vi "Show_raw.00.vi"(3 "t":i32(slide) scale=0.0..1.0, 4 "z":i32(slide) scale=0.0..60.0, 5 "file (use dialog)":path) -> (0 "data 4d":dbl[][][][](array[numeric]), 1 "data 3d":dbl[][][](array[numeric]), 2 "data 2d":dbl[][](array[numeric]))   [LabVIEW 2014]
uses:
  <vilib>/picture/picture.llb/Draw True-Color Pixmap.vi
panel:
  in  "color":enum16{"gray", "color"}(ring)
  in  "Bright":dbl(knob)=512.0 scale=-500.0..500.0
  out "pixel size":sgl[](array[numeric])
  in  "Constrast":dbl(knob)=512.0 scale=0.0..2000.0
  in  "State":bool
  out "2D Picture":picture
  in  "Zoom Factor":sgl=5.0
  out "size(s) 3":i32[](array[numeric])
  out "datatype":string
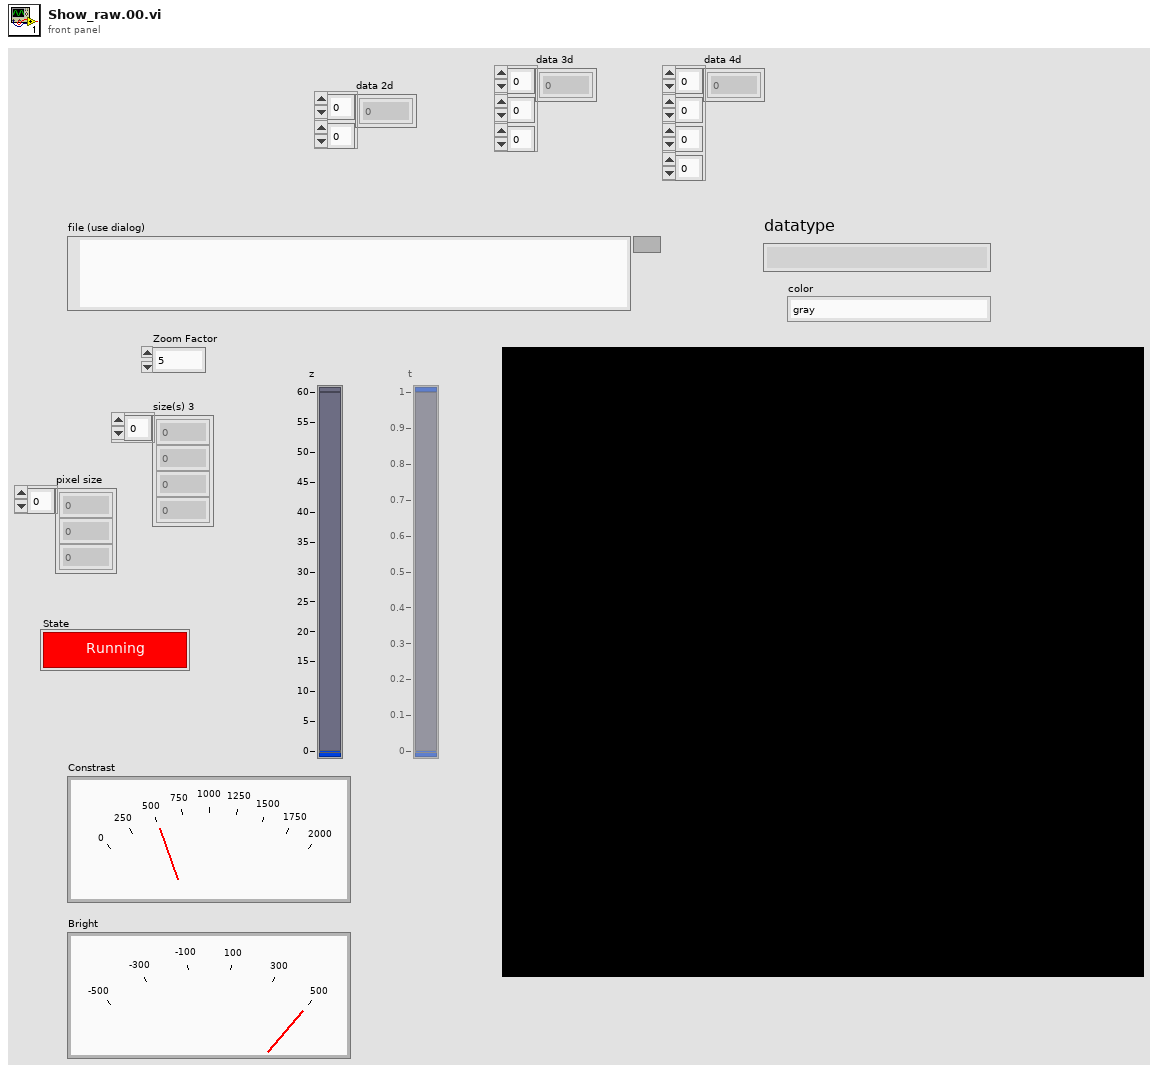
[diagram p1: front panel]
types:
  T1 = enum8{"Enabled", "Disabled", "Disabled and Grayed Out"}
  T2 = typedef "head_data.ctl" = cluster{"hdr size":i32, "dim":i32[], "data bit size":i32, "datatype":string, "pixel size ":sgl[], "voxel offset":sgl, "range of calibration values-max,min":sgl[], " pixel values- max, min":sgl[], "slice orientation":u16}
  T3 = enum32{"Invalid", "Standard", "Closed", "Hidden", "Minimized", "Maximized"}
  T4 = typedef "imagedata.ctl" = cluster{"image type":i32, "image depth":i32, "image":u8[], "mask":u8[], "colors":u32[], "Rectangle":cluster{"left":i16, "top":i16, "right":i16, "bottom":i16}}
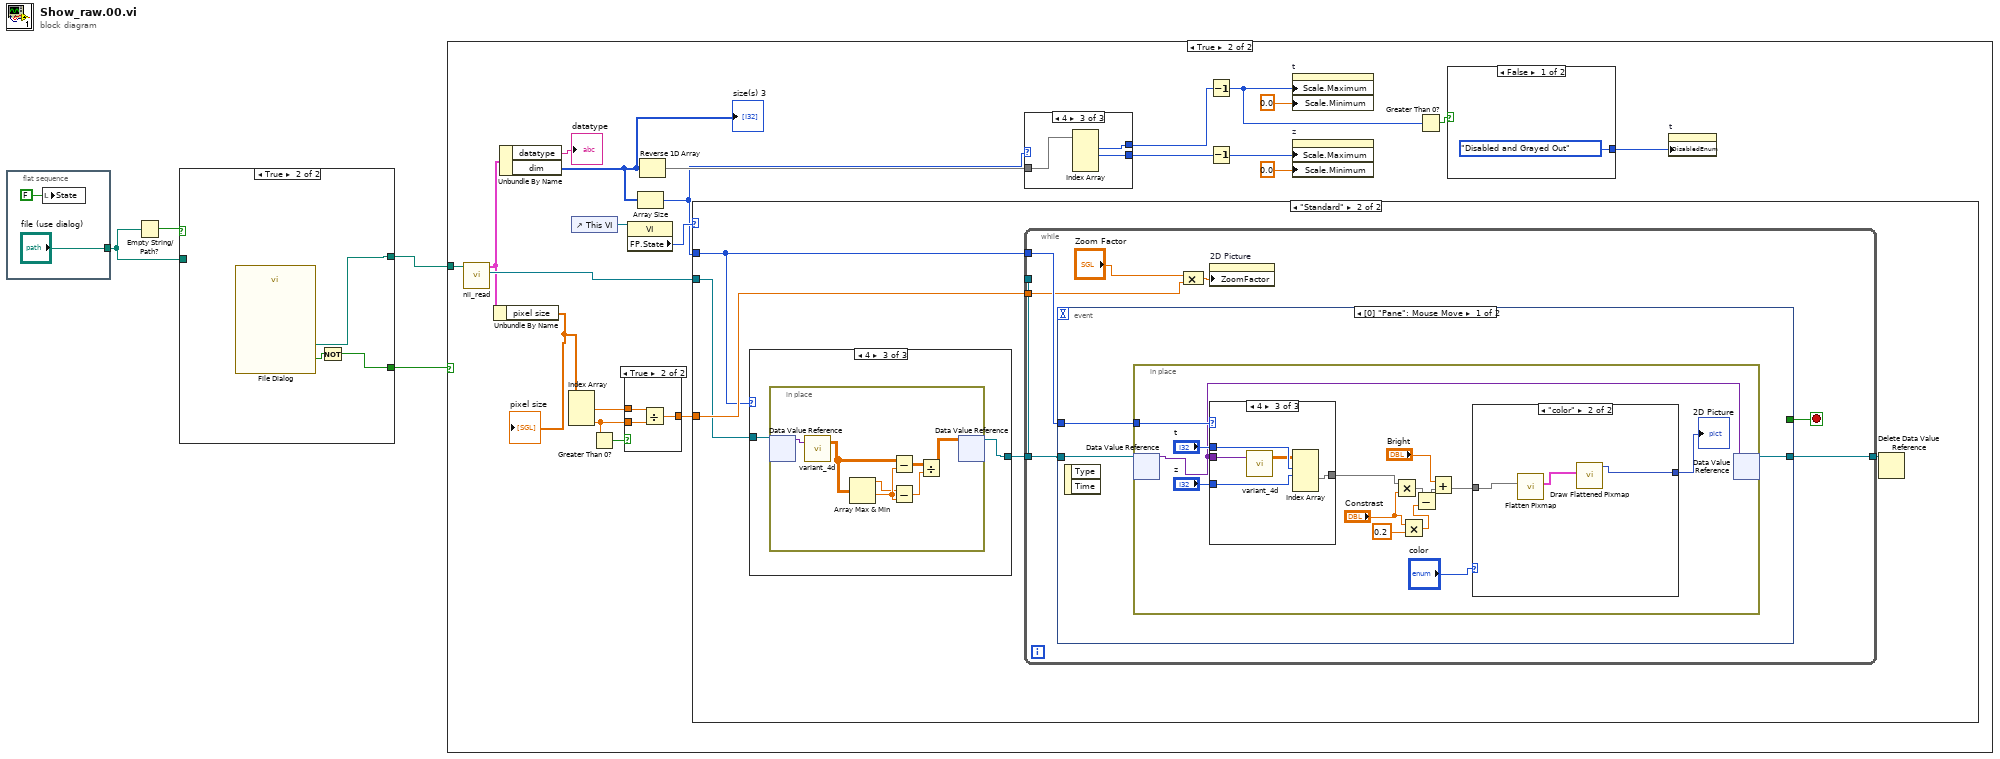
[diagram p0: block diagram]
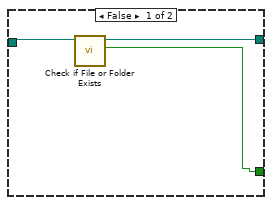
[diagram p2: hidden frame]
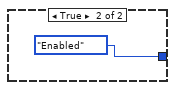
[diagram p4: hidden frame]
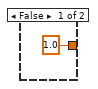
[diagram p5: hidden frame]
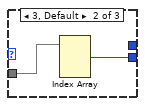
[diagram p7: hidden frame]
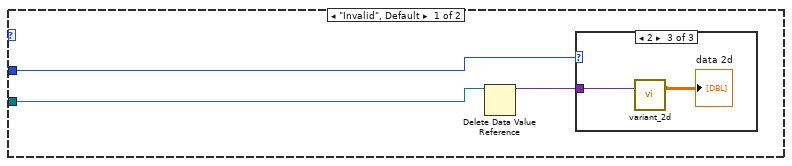
[diagram p8: hidden frame]
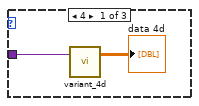
[diagram p9: hidden frame]
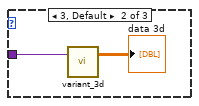
[diagram p10: hidden frame]
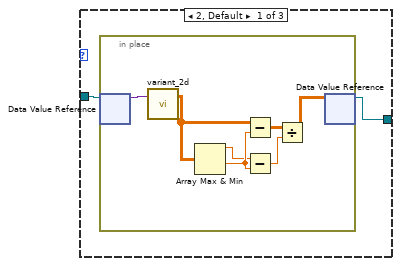
[diagram p11: hidden frame]
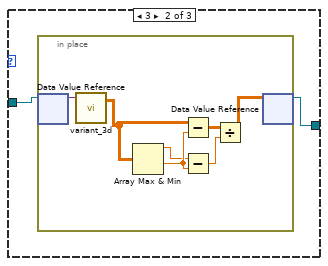
[diagram p12: hidden frame]
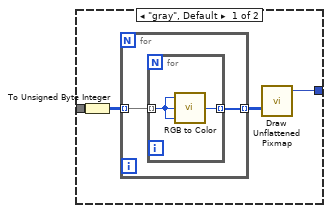
[diagram p13: hidden frame]
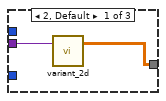
[diagram p14: hidden frame]
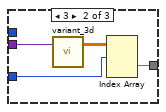
[diagram p15: hidden frame]
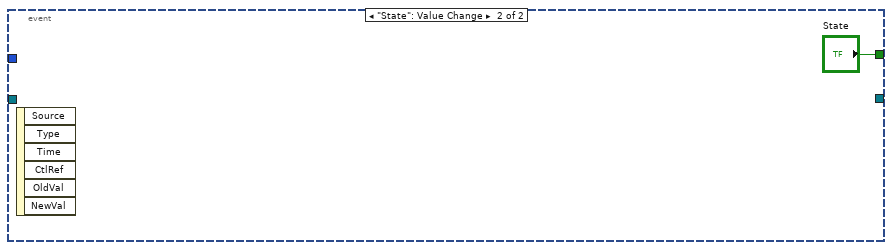
[diagram p16: hidden frame]
diagram:
  n1 = flat-sequence {
    tunnel: ["file (use dialog)"] -> w4
    frame #0 {
      n2 = local write "State"(FALSE ("stop")) -> ()
    }
  }
  n3 = Empty String/Path?(string/path=w4) -> (empty?=w3:bool)
  n4 = case shown="True" w3 {
    tunnel: w4 -> [w9 _]
    tunnel: [w7 w12] -> w1
    tunnel: [w8 w10] -> w2
    frame False {
      n5 = call <vilib>:"Check if File or Folder Exists.vi"("path"=w9) -> ("file or folder exists?"=w7:bool, "dup path"=w8:path)  [unwired: 8 in, 1 out]
    }
    frame True {
      n6 = call "File Dialog"() -> ("selected path"=w10:path, "cancelled"=w11:bool)  [unwired: 12 in, 2 out]
      n7 = Not(x=w11) -> (.not. x?=w12:bool)
    }
  }
  n8 = case shown="True" w1 {
    tunnel: w2 -> [_ w29]
    frame False {
    }
    frame True {
      n9 = call "nii_read.vi"("file (use dialog)"=w29) -> ("data value reference"=w32:refnum<data-value>, "Data"=w22:T2)  [unwired: 6 in, 3 out]
      n10 = Unbundle By Name(w22) -> ("pixel size"=w21:sgl[])
      "pixel size" <- w21
      n11 = Unbundle By Name(w22) -> ("datatype"=→"datatype":string, "dim"=w16:i32[])
      "size(s) 3" <- w16
      n12 = Index Array(array=w21) -> (element #1=w20:sgl, element #3=w19:sgl)  [unwired: 3 in, 1 out]
      n13 = control-ref of="This VI"() -> (w33:refnum<vi>)
      n14 = Greater Than 0?(x=w19) -> (x > 0?=w18:bool)
      n15 = case shown="True" w18 {
        tunnel: w19 -> [_ w38]
        tunnel: w20 -> [_ w40]
        tunnel: [sgl 1.0 w39] -> w17
        frame False {
        }
        frame True {
          n16 = Divide(x=w40, y=w38) -> (x/y=w39:sgl)
        }
      }
      n17 = property class="VI"(reference=w33) -> ("FP.State"=w31:T3)  [unwired: 1 in, 2 out]
      n18 = Array Size(array=w16) -> (size(s)=w26:i32)
      n19 = Reverse 1D Array(array=w16) -> (reversed array=w30:i32[])
      n20 = case shown="\"Standard\"" w31 {
        tunnel: w32 -> [w48 w56]
        tunnel: w26 -> [w47 w57]
        tunnel: w17 -> [_ w59]
        frame "Invalid", Default {
          n21 = Delete Data Value Reference(data value reference=w48) -> (data value=w46:variant)  [unwired: 1 in, 1 out]
          n22 = case shown="2" w47 {
            tunnel: w46 -> [w50 w52 w54]
            frame 4 {
              n23 = call "variant_4d.vi"("variant"=w50) -> ("data"=→"data 4d":dbl[][][][])  [unwired: 2 in]
            }
            frame 3, Default {
              n24 = call "variant_3d.vi"("variant"=w52) -> ("data"=→"data 3d":dbl[][][])  [unwired: 2 in]
            }
            frame 2 {
              n25 = call "variant_2d.vi"("variant"=w54) -> ("data"=→"data 2d":dbl[][])  [unwired: 2 in]
            }
          }
        }
        frame "Standard" {
          n26 = case shown="4" w57 {
            tunnel: w56 -> [w61 w70 w79]
            tunnel: [w60 w69 w78] -> w55
            frame 2, Default {
              n27 = in-place {
                n28 = in-place-dvr #1(w61) -> (w63:variant)  [unwired: 1 out]
                n29 = call "variant_2d.vi"("variant"=w63) -> ("data"=w64:dbl[][])  [unwired: 2 in]
                n30 = Array Max & Min(array=w64) -> (max value=w65:dbl, min value=w66:dbl)  [unwired: 2 out]
                n31 = Subtract(x=w64, y=w66) -> (x-y=w68:dbl[][])
                n32 = Subtract(x=w65, y=w66) -> (x-y=w67:dbl)
                n33 = Divide(x=w68, y=w67) -> (x/y=w62:dbl[][])
                n34 = in-place-dvr #1(w62) -> (w60:refnum<data-value>)  [unwired: 1 out]
              }
            }
            frame 3 {
              n35 = in-place {
                n36 = in-place-dvr #2(w70) -> (w72:variant)  [unwired: 1 out]
                n37 = call "variant_3d.vi"("variant"=w72) -> ("data"=w71:dbl[][][])  [unwired: 2 in]
                n38 = Array Max & Min(array=w71) -> (max value=w74:dbl, min value=w75:dbl)  [unwired: 2 out]
                n39 = Subtract(x=w71, y=w75) -> (x-y=w77:dbl[][][])
                n40 = Subtract(x=w74, y=w75) -> (x-y=w76:dbl)
                n41 = Divide(x=w77, y=w76) -> (x/y=w73:dbl[][][])
                n42 = in-place-dvr #2(w73) -> (w69:refnum<data-value>)  [unwired: 1 out]
              }
            }
            frame 4 {
              n43 = in-place {
                n44 = in-place-dvr #3(w79) -> (w81:variant)  [unwired: 1 out]
                n45 = call "variant_4d.vi"("variant"=w81) -> ("data"=w80:dbl[][][][])  [unwired: 2 in]
                n46 = Array Max & Min(array=w80) -> (max value=w83:dbl, min value=w84:dbl)  [unwired: 2 out]
                n47 = Subtract(x=w80, y=w84) -> (x-y=w86:dbl[][][][])
                n48 = Subtract(x=w83, y=w84) -> (x-y=w85:dbl)
                n49 = Divide(x=w86, y=w85) -> (x/y=w82:dbl[][][][])
                n50 = in-place-dvr #3(w82) -> (w78:refnum<data-value>)  [unwired: 1 out]
              }
            }
          }
          n51 = while {
            tunnel: [w87] -> _
            tunnel: w57 -> [w92]
            tunnel: w59 -> [w89]
            tunnel: [w88] -> w58
            tunnel: w55 -> [w87]
            stop <- w93 stop-if-true
            n52 = event shown="[0] \"Pane\": Mouse Move" {
              selector: _ -> [_ _]
              dyn-events: _ -> [_ _]
              timeout: _ -> [_ _]
              tunnel: [_ "State"] -> w93
              tunnel: w87 -> [w95 _]
              tunnel: w92 -> [w96 _]
              tunnel: [w94 _] -> w88
              event Mouse Move {
                n53 = event-data() -> ()  [unwired: 1 in, 2 out]
                n54 = in-place {
                  in-place-border: w96 -> [w110]
                  n55 = in-place-dvr #4(w95) -> (w107:variant)  [unwired: 1 out]
                  n56 = case shown="4" w110 {
                    tunnel: [w122 w127 w131] -> w105
                    tunnel: "z" -> [_ w125 w129]
                    tunnel: w107 -> [w123 w126 w132]
                    tunnel: "t" -> [_ _ w130]
                    frame 2, Default {
                      n57 = call "variant_2d.vi"("variant"=w123) -> ("data"=w122:dbl[][])  [unwired: 2 in]
                    }
                    frame 3 {
                      n58 = call "variant_3d.vi"("variant"=w126) -> ("data"=w124:dbl[][][])  [unwired: 2 in]
                      n59 = Index Array(array=w124, index (dim 0)=w125) -> (element=w127:dbl[][])  [unwired: 2 in]
                    }
                    frame 4 {
                      n60 = call "variant_4d.vi"("variant"=w132) -> ("data"=w128:dbl[][][][])  [unwired: 2 in]
                      n61 = Index Array(array=w128, index (dim 0)=w130, index (dim 1)=w129) -> (element=w131:dbl[][])  [unwired: 2 in]
                    }
                  }
                  n62 = Multiply(x=w105, y="Constrast") -> (x*y=w103:dbl[][])
                  n63 = Multiply(x="Constrast", y=0.2) -> (x*y=w100:dbl)
                  n64 = Subtract(x=w103, y=w100) -> (x-y=w99:dbl[][])
                  n65 = Add(x="Bright", y=w99) -> (x+y=w104:dbl[][])
                  n66 = case shown="\"color\"" "color" {
                    tunnel: w104 -> [w113 w121]
                    tunnel: [w111 w119] -> w97
                    frame "gray", Default {
                      n67 = To Unsigned Byte Integer(number=w113) -> (unsigned 8bit integer=w114:u8[][])
                      n68 = for {
                        tunnel: w114 -> [w116] mode=indexing
                        tunnel: [w115] -> w112 mode=indexing
                        n69 = for {
                          tunnel: w116 -> [w117] mode=indexing
                          tunnel: [w118] -> w115 mode=indexing
                          n70 = call <vilib>:"RGB to Color.vi"("B"=w117, "G"=w117, "R"=w117) -> ("Color"=w118:u32)
                        }
                      }
                      n71 = call-poly <vilib>:"Draw Unflattened Pixmap.vi"("data (RGB format)"=w112) -> ("new picture"=w111:picture)  [unwired: 8 in]
                    }
                    frame "color" {
                      n72 = call <vilib>:"Flatten Pixmap.vi"("8-bit pixmap"=w121) -> ("image data"=w120:T4)  [unwired: 10 in]
                      n73 = call <vilib>:"Draw Flattened Pixmap.vi"("image data"=w120) -> ("new picture"=w119:picture)  [unwired: 8 in]
                    }
                  }
                  "2D Picture" <- w97
                  n74 = in-place-dvr #4(w107) -> (w94:refnum<data-value>)  [unwired: 1 out]
                }
              }
              event "State": Value Change {
                n75 = event-data() -> ()  [unwired: 1 in, 6 out]
              }
            }
            n76 = Compound Arithmetic op=MULTIPLY("Zoom Factor", w89) -> (w91:sgl)
            n77 = property on="2D Picture" class="Pict"("ZoomFactor"=w91) -> ()  [unwired: 2 in, 2 out]
          }
          n78 = Delete Data Value Reference(data value reference=w58) -> ()  [unwired: 1 in, 2 out]
        }
      }
      n79 = case shown="4" w26 {
        tunnel: w30 -> [_ w42 w45]
        tunnel: [_ _ w44] -> w28
        tunnel: [_ w41 w43] -> w27
        frame 2 {
        }
        frame 3, Default {
          n80 = Index Array(array=w42) -> (element #1=w41:i32)  [unwired: 3 in, 2 out]
        }
        frame 4 {
          n81 = Index Array(array=w45) -> (element #1=w44:i32, element #2=w43:i32)  [unwired: 4 in, 2 out]
        }
      }
      n82 = Decrement(x=w28) -> (x-1=w14:i32)
      n83 = Decrement(x=w27) -> (x-1=w25:i32)
      n84 = property on="t" class="Slide (strict)"("Scale.Maximum"=w14, "Scale.Minimum"=0.0 ("Scale.Range:Minimum")) -> ()  [unwired: 2 in, 2 out]
      n85 = property on="z" class="Slide (strict)"("Scale.Maximum"=w25, "Scale.Minimum"=0.0 ("Scale.Range:Minimum")) -> ()  [unwired: 2 in, 2 out]
      n86 = Greater Than 0?(x=w14) -> (x > 0?=w15:bool)
      n87 = case shown="False" w15 {
        tunnel: [T1."Disabled and Grayed Out" ("Disabled") T1."Enabled" ("Disabled")] -> w13
        frame False {
        }
        frame True {
        }
      }
      n88 = property on="t" class="Slide (strict)"("DisabledEnum"=w13) -> ()  [unwired: 2 in, 2 out]
    }
  }
